vi "Frisbee Counter.vi"   [LabVIEW 2012]
uses:
  BotStatus.vi
types:
  T1 = cluster{"Middle":bool, "InFlipper":bool, "Bottom":bool, "FlipperDown":bool, "Frizbee Counter":dbl}
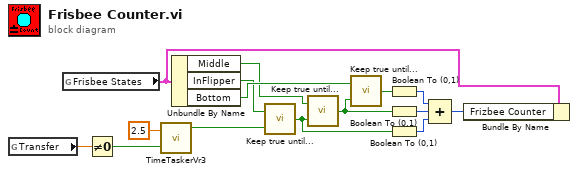
[diagram p0: block diagram]
diagram:
  n1 = global read "BotStatus.vi" "Transfer"() -> (w11:dbl)
  n2 = global read "BotStatus.vi" "Frisbee States"() -> (w8:T1)
  n3 = Not Equal To 0?(x=w11) -> (x != 0?=w12:bool)
  n4 = call "TimeTaskerVr3.vi"("Delay(sec)"=2.5, "Start Counting?"=w12) -> ("TimePast?"=w13:bool)  [unwired: 2 out]
  n5 = Unbundle By Name(w8) -> ("Middle"=w9:bool, "InFlipper"=w10:bool, "Bottom"=w15:bool)
  n6 = call "Keep true until....vi"("Changer"=w13, "Keep"=w10) -> ("Value"=w1:bool)
  n7 = call "Keep true until....vi"("Changer"=w1, "Keep"=w9) -> ("Value"=w2:bool)
  n8 = call "Keep true until....vi"("Changer"=w2, "Keep"=w15) -> ("Value"=w3:bool)
  n9 = Boolean To (0,1)(Boolean=w3) -> (0, 1=w4:i16)
  n10 = Boolean To (0,1)(Boolean=w2) -> (0, 1=w6:i16)
  n11 = Boolean To (0,1)(Boolean=w1) -> (0, 1=w5:i16)
  n12 = Compound Arithmetic op=ADD(w4, w6, w5) -> (w7:i16)
  n13 = Bundle By Name(cluster=w8, "Frizbee Counter"=w7) -> ()  [unwired: 1 out]
